vi "main.vi"() -> ()   [LabVIEW 2023]
uses:
  #typedef_data.ctl
panel:
  out "result":dbl
  in  "Data":T1
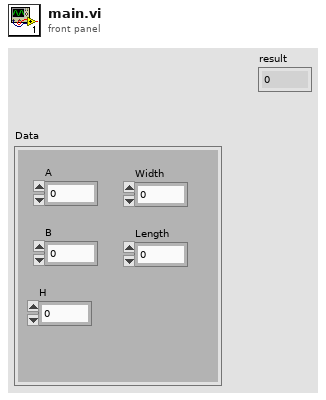
[diagram p1: front panel]
types:
  T1 = typedef "#typedef_data.ctl" = cluster{"A":dbl, "B":dbl, "H":dbl, "Width":dbl, "Length":dbl}
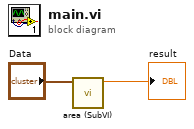
[diagram p0: block diagram]
diagram:
  n1 = call "area (SubVI).vi"("Data"="Data") -> ("Numeric"=→"result":dbl)  [unwired: 9 in, 1 out]
